vi "SOUR_POW_LEV_SLOP_STAT.vi"(0 "VISA IN":refnum<visa-resource-name>, 1 "Slope ON/OFF":bool, 5 "error in":errorcluster, 7 "Channel":i32) -> (14 "VISA Out":refnum<visa-resource-name>, 19 "error out":errorcluster)   [LabVIEW 2018, in "PNA-X.lvlib"]
doc: "SOURce<cnum>:POWer[:LEVel]:SLOPe:STATe <ON | OFF> \n(Read-Write) Turns Power Slope ON or OFF. \nParameters \n<cnum> Any existing channel number. If unspecified, value is set to 1 \n<ON|OFF> ON (or 1) - turns slope ON. \nOFF (or 0) - turns slope OFF. \nExamples SOUR:POW:SLOP:STAT ON \nsource2:power:slope:state off \nQuery Syntax SOURce<cnum>:POWer[:LEVel]:SLOPe:STATe? \nReturn Type Boolean (1 = ON, 0 = OFF) \nDefault OFF"
uses:
  PNA-X.lvlib
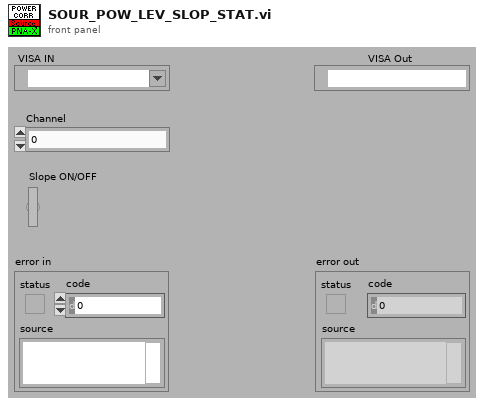
[diagram p1: front panel]
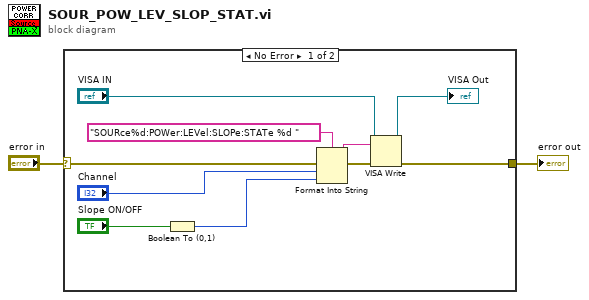
[diagram p0: block diagram]
diagram:
  n1 = case shown="No Error" "error in" {
    selector: "error in" -> [w12 w13]
    tunnel: [w7 w13] -> w1
    frame No Error {
      n2 = Boolean To (0,1)(Boolean="Slope ON/OFF") -> (0, 1=w3:i16)
      n3 = Format Into String(format string="SOURce%d:POWer:LEVel:SLOPe:STATe %d " ("Cmdline"), error in=w12, "Channel", w3) -> (resulting string=w10:string, error out=w11:errorcluster)  [unwired: 1 in]
      n4 = VISA Write(VISA resource name="VISA IN", write buffer=w10, error in (no error)=w11) -> (VISA resource name out=→"VISA Out":refnum<visa-resource-name>, error out=w7:errorcluster)  [unwired: 1 out]
    }
    frame Error {
    }
  }
  "error out" <- w1
